vi "allocate cache.vi"(10 "scans per write":i32, 11 "counts":T1[](array[typedef])) -> (3 "cache allocation":T3)   [LabVIEW 2013, in "TDMS datalogger runtime.lvclass"]
uses:
  TDMS datalogger runtime.lvclass
  data cache.ctl
  <vilib>/NI/Tag Bus/table/allocation specification.ctl
  <vilib>/NI/Tag Bus/tag/Data Type.ctl
  <vilib>/NI/Tag Bus/tag/tag descriptor.lvclass
  <vilib>/NI/Tag Bus/table/data table.lvlib
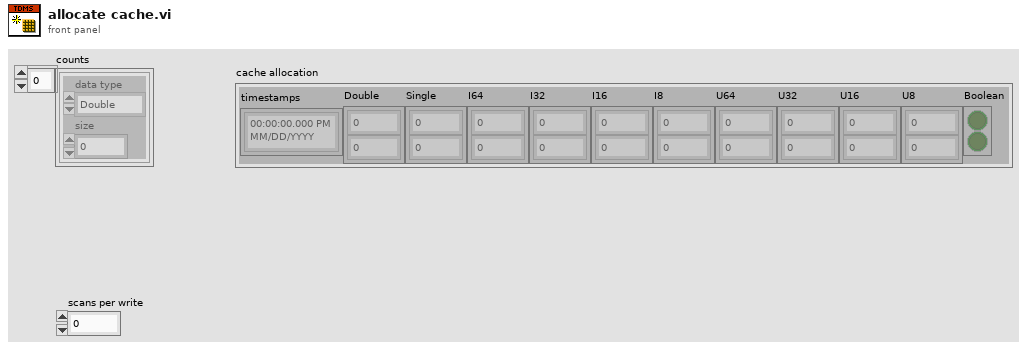
[diagram p1: front panel]
types:
  T1 = typedef "tag bus.lvlib/data table.lvlib/allocation specification.ctl" = cluster{"data type":T2, "size":i32}
  T2 = typedef "tag bus.lvlib/tag descriptor.lvclass/Data Type.ctl" = enum16{"Double", "Single", "I64", "I32", "I16", "I8", "U64", "U32", "U16", "U8", "Boolean", "String", "Array of Double", "Array of Single", "Array of I64", "Array of I32", "Array of I16", "Array of I8", "Array of U64", "Array of U32", "Array of U16", "Array of U8", "Array of Boolean", "Array of String"}
  T3 = typedef "TDMS datalogger runtime.lvclass/data cache.ctl" = cluster{"timestamps":timestamp[], "Double":dbl[][], "Single":sgl[][], "I64":i64[][], "I32":i32[][], "I16":i16[][], "I8":i8[][], "U64":u64[][], "U32":u32[][], "U16":u16[][], "U8":u8[][], "Boolean":bool[][]}
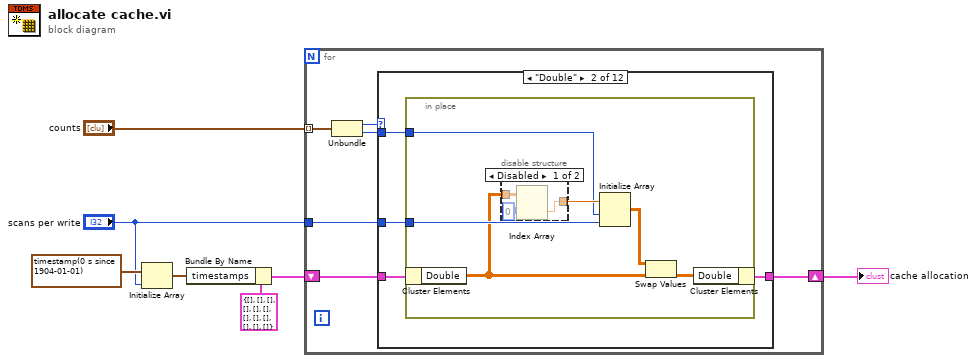
[diagram p0: block diagram]
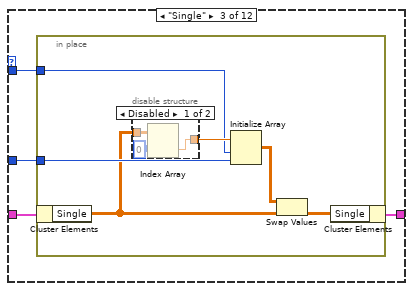
[diagram p4: hidden frame]
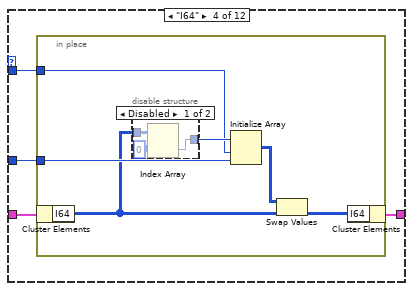
[diagram p6: hidden frame]
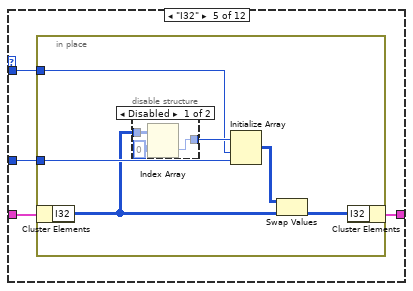
[diagram p8: hidden frame]
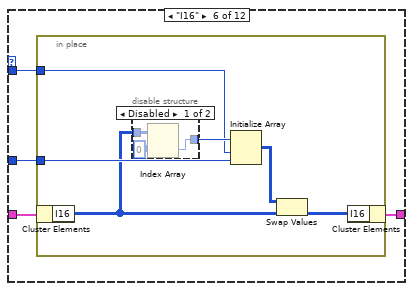
[diagram p10: hidden frame]
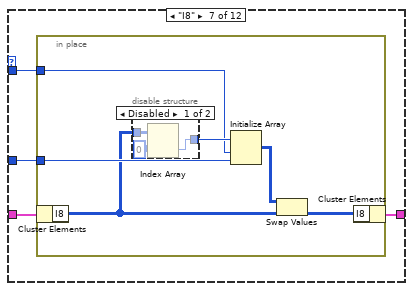
[diagram p12: hidden frame]
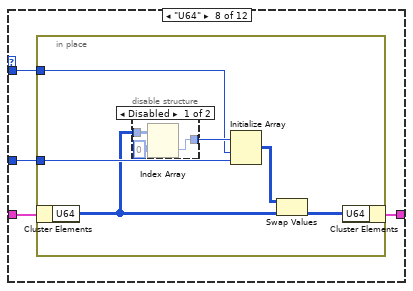
[diagram p14: hidden frame]
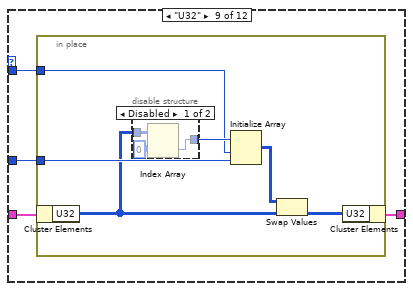
[diagram p16: hidden frame]
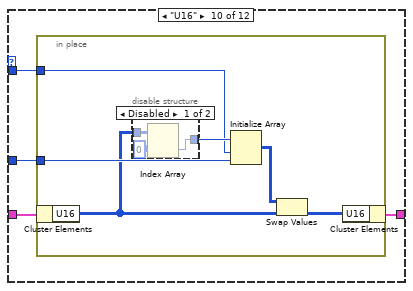
[diagram p18: hidden frame]
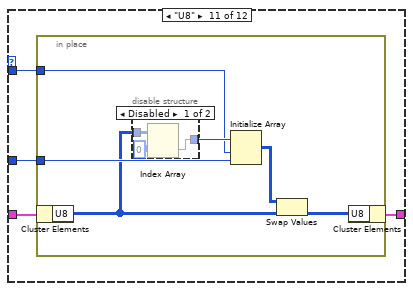
[diagram p20: hidden frame]
diagram:
  n1 = Initialize Array(timestamp(0 s since 1904-01-01), "scans per write") -> (w2:timestamp[])
  n2 = Bundle By Name(cluster=T3 {"timestamps"=[], "Double"=[], "Single"=[], "I64"=[], "I32"=[], "I16"=[], "I8"=[], "U64"=[], "U32"=[], "U16"=[], "U8"=[], "Boolean"=[]} ("cache allocation"), "timestamps"=w2) -> (w4:T3)
  n3 = for {
    shift-right: [w9] -> w6
    shift-left: w4 -> [w10]
    tunnel: "counts" -> [w13] mode=indexing
    tunnel: "scans per write" -> [w8]
    n4 = Unbundle(w13) -> ("data type"=w12:T2, "size"=w11:i32)
    n5 = case shown="\"Double\"" w12 {
      tunnel: w11 -> [_ w15 w28 w41 w54 w67 w80 w93 w106 w119 w132 w145]
      tunnel: w10 -> [w14 w18 w31 w44 w57 w70 w83 w96 w109 w122 w135 w148]
      tunnel: [w14 w17 w30 w43 w56 w69 w82 w95 w108 w121 w134 w147] -> w9
      tunnel: w8 -> [_ w16 w29 w42 w55 w68 w81 w94 w107 w120 w133 w146]
      frame Default {
      }
      frame "Double" {
        n6 = in-place {
          in-place-border: w16 -> [w24]
          in-place-border: w15 -> [w22]
          n7 = in-place-cluster #1(w18) -> ("Double"=w21:dbl[][])
          n8 = disable-structure shown="Disabled" {
            disable-tunnel: w21 -> [w27 _]
            disable-tunnel: [w25 _] -> w23
            frame Disabled {
              w26 = 0 ("disabled index (col)")
              n9 = Index Array(array=w27, index (row)=w26, index (col)=w26) -> (element=w25:dbl)
            }
            frame Enabled {
            }
          }
          n10 = Initialize Array(w23, w22, w24) -> (w19:dbl[][])
          n11 = Swap Values(12:w19, 14:w21) -> (3:w20:dbl[][])  [unwired: 1 in, 1 out]
          n12 = in-place-cluster #1("Double"=w20) -> (w17:T3)
        }
      }
      frame "Single" {
        n13 = in-place {
          in-place-border: w29 -> [w37]
          in-place-border: w28 -> [w35]
          n14 = in-place-cluster #2(w31) -> ("Single"=w34:sgl[][])
          n15 = disable-structure shown="Disabled" {
            disable-tunnel: w34 -> [w40 _]
            disable-tunnel: [w38 _] -> w36
            frame Disabled {
              w39 = 0 ("disabled index (col)")
              n16 = Index Array(array=w40, index (row)=w39, index (col)=w39) -> (element=w38:sgl)
            }
            frame Enabled {
            }
          }
          n17 = Initialize Array(w36, w35, w37) -> (w32:sgl[][])
          n18 = Swap Values(12:w32, 14:w34) -> (3:w33:sgl[][])  [unwired: 1 in, 1 out]
          n19 = in-place-cluster #2("Single"=w33) -> (w30:T3)
        }
      }
      frame "I64" {
        n20 = in-place {
          in-place-border: w42 -> [w50]
          in-place-border: w41 -> [w48]
          n21 = in-place-cluster #3(w44) -> ("I64"=w47:i64[][])
          n22 = disable-structure shown="Disabled" {
            disable-tunnel: w47 -> [w53 _]
            disable-tunnel: [w51 _] -> w49
            frame Disabled {
              w52 = 0 ("disabled index (col)")
              n23 = Index Array(array=w53, index (row)=w52, index (col)=w52) -> (element=w51:i64)
            }
            frame Enabled {
            }
          }
          n24 = Initialize Array(w49, w48, w50) -> (w45:i64[][])
          n25 = Swap Values(12:w45, 14:w47) -> (3:w46:i64[][])  [unwired: 1 in, 1 out]
          n26 = in-place-cluster #3("I64"=w46) -> (w43:T3)
        }
      }
      frame "I32" {
        n27 = in-place {
          in-place-border: w55 -> [w63]
          in-place-border: w54 -> [w61]
          n28 = in-place-cluster #4(w57) -> ("I32"=w60:i32[][])
          n29 = disable-structure shown="Disabled" {
            disable-tunnel: w60 -> [w66 _]
            disable-tunnel: [w64 _] -> w62
            frame Disabled {
              w65 = 0 ("disabled index (col)")
              n30 = Index Array(array=w66, index (row)=w65, index (col)=w65) -> (element=w64:i32)
            }
            frame Enabled {
            }
          }
          n31 = Initialize Array(w62, w61, w63) -> (w58:i32[][])
          n32 = Swap Values(12:w58, 14:w60) -> (3:w59:i32[][])  [unwired: 1 in, 1 out]
          n33 = in-place-cluster #4("I32"=w59) -> (w56:T3)
        }
      }
      frame "I16" {
        n34 = in-place {
          in-place-border: w68 -> [w76]
          in-place-border: w67 -> [w74]
          n35 = in-place-cluster #5(w70) -> ("I16"=w73:i16[][])
          n36 = disable-structure shown="Disabled" {
            disable-tunnel: w73 -> [w79 _]
            disable-tunnel: [w77 _] -> w75
            frame Disabled {
              w78 = 0 ("disabled index (col)")
              n37 = Index Array(array=w79, index (row)=w78, index (col)=w78) -> (element=w77:i16)
            }
            frame Enabled {
            }
          }
          n38 = Initialize Array(w75, w74, w76) -> (w71:i16[][])
          n39 = Swap Values(12:w71, 14:w73) -> (3:w72:i16[][])  [unwired: 1 in, 1 out]
          n40 = in-place-cluster #5("I16"=w72) -> (w69:T3)
        }
      }
      frame "I8" {
        n41 = in-place {
          in-place-border: w81 -> [w89]
          in-place-border: w80 -> [w87]
          n42 = in-place-cluster #6(w83) -> ("I8"=w86:i8[][])
          n43 = disable-structure shown="Disabled" {
            disable-tunnel: w86 -> [w92 _]
            disable-tunnel: [w90 _] -> w88
            frame Disabled {
              w91 = 0 ("disabled index (col)")
              n44 = Index Array(array=w92, index (row)=w91, index (col)=w91) -> (element=w90:i8)
            }
            frame Enabled {
            }
          }
          n45 = Initialize Array(w88, w87, w89) -> (w84:i8[][])
          n46 = Swap Values(12:w84, 14:w86) -> (3:w85:i8[][])  [unwired: 1 in, 1 out]
          n47 = in-place-cluster #6("I8"=w85) -> (w82:T3)
        }
      }
      frame "U64" {
        n48 = in-place {
          in-place-border: w94 -> [w102]
          in-place-border: w93 -> [w100]
          n49 = in-place-cluster #7(w96) -> ("U64"=w99:u64[][])
          n50 = disable-structure shown="Disabled" {
            disable-tunnel: w99 -> [w105 _]
            disable-tunnel: [w103 _] -> w101
            frame Disabled {
              w104 = 0 ("disabled index (col)")
              n51 = Index Array(array=w105, index (row)=w104, index (col)=w104) -> (element=w103:u64)
            }
            frame Enabled {
            }
          }
          n52 = Initialize Array(w101, w100, w102) -> (w97:u64[][])
          n53 = Swap Values(12:w97, 14:w99) -> (3:w98:u64[][])  [unwired: 1 in, 1 out]
          n54 = in-place-cluster #7("U64"=w98) -> (w95:T3)
        }
      }
      frame "U32" {
        n55 = in-place {
          in-place-border: w107 -> [w115]
          in-place-border: w106 -> [w113]
          n56 = in-place-cluster #8(w109) -> ("U32"=w112:u32[][])
          n57 = disable-structure shown="Disabled" {
            disable-tunnel: w112 -> [w118 _]
            disable-tunnel: [w116 _] -> w114
            frame Disabled {
              w117 = 0 ("disabled index (col)")
              n58 = Index Array(array=w118, index (row)=w117, index (col)=w117) -> (element=w116:u32)
            }
            frame Enabled {
            }
          }
          n59 = Initialize Array(w114, w113, w115) -> (w110:u32[][])
          n60 = Swap Values(12:w110, 14:w112) -> (3:w111:u32[][])  [unwired: 1 in, 1 out]
          n61 = in-place-cluster #8("U32"=w111) -> (w108:T3)
        }
      }
      frame "U16" {
        n62 = in-place {
          in-place-border: w120 -> [w128]
          in-place-border: w119 -> [w126]
          n63 = in-place-cluster #9(w122) -> ("U16"=w125:u16[][])
          n64 = disable-structure shown="Disabled" {
            disable-tunnel: w125 -> [w131 _]
            disable-tunnel: [w129 _] -> w127
            frame Disabled {
              w130 = 0 ("disabled index (col)")
              n65 = Index Array(array=w131, index (row)=w130, index (col)=w130) -> (element=w129:u16)
            }
            frame Enabled {
            }
          }
          n66 = Initialize Array(w127, w126, w128) -> (w123:u16[][])
          n67 = Swap Values(12:w123, 14:w125) -> (3:w124:u16[][])  [unwired: 1 in, 1 out]
          n68 = in-place-cluster #9("U16"=w124) -> (w121:T3)
        }
      }
      frame "U8" {
        n69 = in-place {
          in-place-border: w133 -> [w141]
          in-place-border: w132 -> [w139]
          n70 = in-place-cluster #10(w135) -> ("U8"=w138:u8[][])
          n71 = disable-structure shown="Disabled" {
            disable-tunnel: w138 -> [w144 _]
            disable-tunnel: [w142 _] -> w140
            frame Disabled {
              w143 = 0 ("disabled index (col)")
              n72 = Index Array(array=w144, index (row)=w143, index (col)=w143) -> (element=w142:u8)
            }
            frame Enabled {
            }
          }
          n73 = Initialize Array(w140, w139, w141) -> (w136:u8[][])
          n74 = Swap Values(12:w136, 14:w138) -> (3:w137:u8[][])  [unwired: 1 in, 1 out]
          n75 = in-place-cluster #10("U8"=w137) -> (w134:T3)
        }
      }
      frame "Boolean" {
        n76 = in-place {
          in-place-border: w146 -> [w154]
          in-place-border: w145 -> [w152]
          n77 = in-place-cluster #11(w148) -> ("Boolean"=w151:bool[][])
          n78 = disable-structure shown="Disabled" {
            disable-tunnel: w151 -> [w157 _]
            disable-tunnel: [w155 _] -> w153
            frame Disabled {
              w156 = 0 ("disabled index (col)")
              n79 = Index Array(array=w157, index (row)=w156, index (col)=w156) -> (element=w155:bool)
            }
            frame Enabled {
            }
          }
          n80 = Initialize Array(w153, w152, w154) -> (w149:bool[][])
          n81 = Swap Values(12:w149, 14:w151) -> (3:w150:bool[][])  [unwired: 1 in, 1 out]
          n82 = in-place-cluster #11("Boolean"=w150) -> (w147:T3)
        }
      }
    }
  }
  "cache allocation" <- w6
